vi "Read Waveform Array.vi"(8 "error in (no error)":errorcluster, 11 "LHW-WfmData in":refnum<class "LHW-WfmData.lvclass">) -> (0 "error out":errorcluster, 2 "Waveform Array":waveform(dbl)[](array[waveform]), 3 "LHW-WfmData out":refnum<class "LHW-WfmData.lvclass">)   [LabVIEW 2014, in "LHW-Data.lvlib" / "LHW-WfmData.lvclass"]
doc: "Read waveform array from attribute."
uses:
  LHW-WfmData.lvclass
  LHW-WfmData.lvclass/LHW-WfmData.ctl
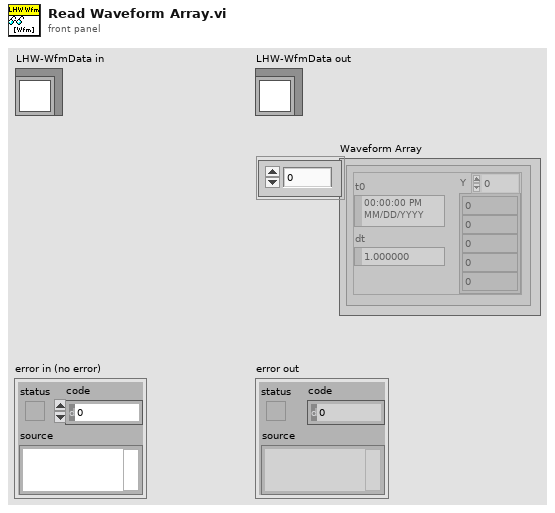
[diagram p1: front panel]
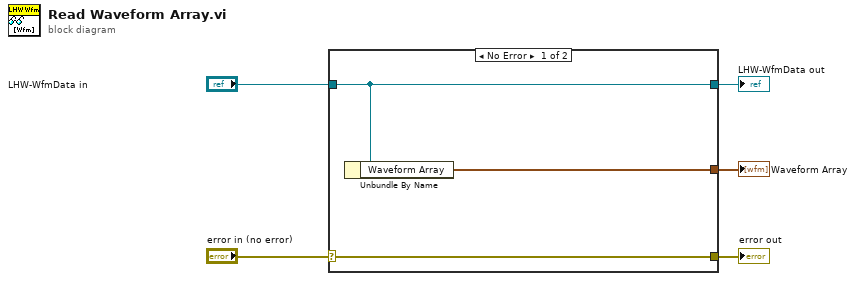
[diagram p0: block diagram]
diagram:
  n1 = case shown="No Error" "error in (no error)" {
    selector: "error in (no error)" -> [w8 w9]
    tunnel: [w8 w9] -> w4
    tunnel: [w7 w10] -> w2
    tunnel: "LHW-WfmData in" -> [w7 w10]
    tunnel: [w6 _] -> w1
    frame No Error {
      n2 = Unbundle By Name(w7) -> ("Waveform Array"=w6:waveform(dbl)[])
    }
    frame Error {
    }
  }
  "error out" <- w4
  "LHW-WfmData out" <- w2
  "Waveform Array" <- w1
